vi "makePoissonDist.vi"(2 "Frequency":dbl=1000.0, 3 "Number of entries in LUT":dbl=2000.0, 4 "Input":dbl) -> (0 "Time to wait (s)":dbl, 1 "Output":u32)   [LabVIEW 2012]
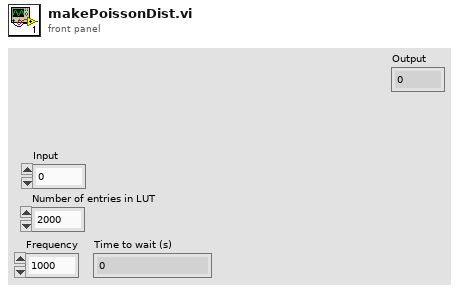
[diagram p1: front panel]
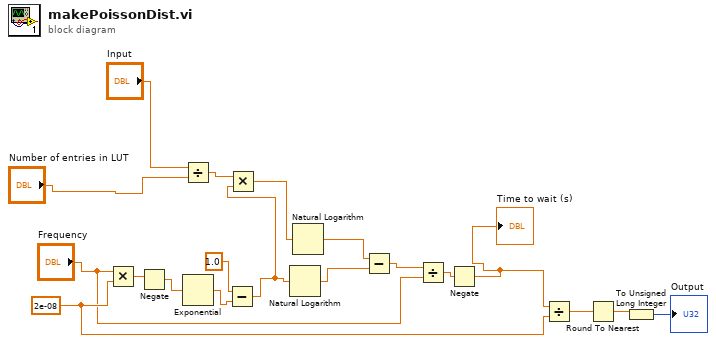
[diagram p0: block diagram]
diagram:
  w19 = 2e-08 ("y")
  n1 = Multiply(x="Frequency", y=w19) -> (x*y=w16:dbl)
  n2 = Negate(x=w16) -> (-x=w15:dbl)
  n3 = Divide(x="Input", y="Number of entries in LUT") -> (x/y=w8:dbl)
  n4 = Exponential(1:w15) -> (0:w13:dbl)
  n5 = Subtract(x=1.0, y=w13) -> (x-y=w7:dbl)
  n6 = Multiply(x=w8, y=w7) -> (x*y=w6:dbl)
  n7 = Natural Logarithm(1:w7) -> (0:w11:dbl)
  n8 = Natural Logarithm(1:w6) -> (0:w12:dbl)
  n9 = Subtract(x=w12, y=w11) -> (x-y=w17:dbl)
  n10 = Divide(x=w17, y="Frequency") -> (x/y=w10:dbl)
  n11 = Negate(x=w10) -> (-x=w9:dbl)
  "Time to wait (s)" <- w9
  n12 = Divide(x=w9, y=w19) -> (x/y=w18:dbl)
  n13 = Round To Nearest(number=w18) -> (nearest integer value=w2:dbl)
  n14 = To Unsigned Long Integer(number=w2) -> (unsigned 32bit integer=→"Output":u32)
